vi "rsidr_core_global.vi"() -> ()   [LabVIEW 2020, in "Rohde&Schwarz RTx Oscilloscopes.lvlib"] (continued)
"Flags"=0, "Help"="Contains attributes for Spectrum Waveform settings."}, {"Level"=3, "Class Only"=FALSE, "Identifier"="RSRTX_ATTR_SPECTRUM_WAVEFORM_ENABLE", "Descriptive Name"="Spectrum Waveform Enable", "Data Type"=3, "Command"="SPEC:WAV:SPEC", "Access"=2, "Range Table"="", "Read Callback"="", "Write Callback"="", "Supported Models"="", "Instrument Options"="", "Flags"=0, "Help"="Enables or diables the indicated waveform.\n\nAvailable Repeated Capabilities:\nNone\n\nRemote-control command(s):\nSPECtrum:WAVeform:SPECtrum[:ENABle]"}, {"Level"=3, "Class Only"=FALSE, "Identifier"="RSRTX_ATTR_SPECTRUM_WAVEFORM_MINIMUM_ENABLE", "Descriptive Name"="Spectrum Waveform Minimum Enable", "Data Type"=3, "Command"="SPEC:WAV:MIN", "Access"=2, "Range Table"="", "Read Callback"="", "Write Callback"="", "Supported Models"="", "Instrument Options"="", "Flags"=0, "Help"="Enables or diables the indicated waveform.\n\nAvailable Repeated Capabilities:\nNone\n\nRemote-control command(s):\nSPECtrum:WAVeform:MINimum[:ENABle]"}, {"Level"=3, "Class Only"=FALSE, "Identifier"="RSRTX_ATTR_SPECTRUM_WAVEFORM_MAXIMUM_ENABLE", "Descriptive Name"="Spectrum Waveform Maximum Enable", "Data Type"=3, "Command"="SPEC:WAV:MAX", "Access"=2, "Range Table"="", "Read Callback"="", "Write Callback"="", "Supported Models"="", "Instrument Options"="", "Flags"=0, "Help"="Enables or diables the indicated waveform.\n\nAvailable Repeated Capabilities:\nNone\n\nRemote-control command(s):\nSPECtrum:WAVeform:MAXimum[:ENABle]"}, {"Level"=3, "Class Only"=FALSE, "Identifier"="RSRTX_ATTR_SPECTRUM_WAVEFORM_AVERAGE_ENABLE", "Descriptive Name"="Spectrum Waveform Average Enable", "Data Type"=3, "Command"="SPEC:WAV:AVER", "Access"=2, "Range Table"="", "Read Callback"="", "Write Callback"="", "Supported Models"="", "Instrument Options"="", "Flags"=0, "Help"="Enables or diables the indicated waveform.\n\nAvailable Repeated Capabilities:\nNone\n\nRemote-control command(s):\nSPECtrum:WAVeform:AVERage[:ENABle]"}, {"Level"=2, "Class Only"=TRUE, "Identifier"="", "Descriptive Name"="Time Domain", "Data Type"=0, "Command"="", "Access"=0, "Range Table"="", "Read Callback"="", "Write Callback"="", "Supported Models"="", "Instrument Options"="", "Flags"=0, "Help"="Contains attributes for Spectrum Time Domain settings."}, {"Level"=3, "Class Only"=FALSE, "Identifier"="RSRTX_ATTR_SPECTRUM_TIME_DOMAIN_POSITION", "Descriptive Name"="Spectrum Time Domain Position", "Data Type"=1, "Command"="SPEC:TIME:POS", "Access"=2, "Range Table"="", "Read Callback"="", "Write Callback"="", "Supported Models"="", "Instrument Options"="", "Flags"=0, "Help"="Sets the time position of the analyzed time range.\n\nAvailable Repeated Capabilities:\nNone\n\nRemote-control command(s):\nSPECtrum:TIME:POSition"}, {"Level"=3, "Class Only"=FALSE, "Identifier"="RSRTX_ATTR_SPECTRUM_TIME_DOMAIN_RANGE", "Descriptive Name"="Spectrum Time Domain Range", "Data Type"=1, "Command"="SPEC:TIME:RANG", "Access"=2, "Range Table"="", "Read Callback"="", "Write Callback"="", "Supported Models"="", "Instrument Options"="", "Flags"=0, "Help"="Sets the time range for the time domain diagram.\n\nAvailable Repeated Capabilities:\nNone\n\nRemote-control command(s):\nSPECtrum:TIME:RANGe"}, {"Level"=1, "Class Only"=TRUE, "Identifier"="", "Descriptive Name"="Digital Voltmeter and Counter", "Data Type"=0, "Command"="", "Access"=0, "Range Table"="", "Read Callback"="", "Write Callback"="", "Supported Models"="", "Instrument Options"="", "Flags"=0, "Help"="Contains attributes for DVM and Counter settings."}, {"Level"=2, "Class Only"=FALSE, "Identifier"="RSRTX_ATTR_DVM_ENABLE", "Descriptive Name"="DVM Enable", "Data Type"=3, "Command"="DVM{DigitalVoltmeter}:ENAB", "Access"=2, "Range Table"="", "Read Callback"="", "Write Callback"="", "Supported Models"="", "Instrument Options"="", "Flags"=0, "Help"="Enables and disables all configured voltmeter measurements.\n\nAvailable Repeated Capabilities:\nDigitalVoltmeter: DVM1, DVM2, DVM3, DVM4\r\n\nRemote-control command(s):\nDVM<m>:ENABle"}, {"Level"=2, "Class Only"=FALSE, "Identifier"="RSRTX_ATTR_DVM_SOURCE", "Descriptive Name"="DVM Source", "Data Type"=0, "Command"="DVM{DigitalVoltmeter}:SOUR", "Access"=2, "Range Table"="rsrtx_rngSource", "Read Callback"="", "Write Callback"="", "Supported Models"="", "Instrument Options"="", "Flags"=0, "Help"="Sets the measurement source for the indicated DVM measurement.\n\nAvailable Repeated Capabilities:\nDigitalVoltmeter: DVM1, DVM2, DVM3, DVM4\r\n\nRemote-control command(s):\nDVM<m>:SOURce"}, {"Level"=2, "Class Only"=FALSE, "Identifier"="RSRTX_ATTR_DVM_TYPE", "Descriptive Name"="DVM Type", "Data Type"=0, "Command"="DVM{DigitalVoltmeter}:TYPE", "Access"=2, "Range Table"="RsRtx_rngDVMType", "Read Callback"="", "Write Callback"="", "Supported Models"="", "Instrument Options"="", "Flags"=0, "Help"="Sets the measurement type for the indicated DVM measurement.\nSet OFF to disable the measurement.\n\nAvailable Repeated Capabilities:\nDigitalVoltmeter: DVM1, DVM2, DVM3, DVM4\r\n\nRemote-control command(s):\nDVM<m>:TYPE"}, {"Level"=2, "Class Only"=FALSE, "Identifier"="RSRTX_ATTR_DVM_POSITION", "Descriptive Name"="DVM Position", "Data Type"=0, "Command"="DVM{DigitalVoltmeter}:POS", "Access"=2, "Range Table"="RsRtx_rngDVMPosition", "Read Callback"="", "Write Callback"="", "Supported Models"="", "Instrument Options"="", "Flags"=0, "Help"="Sets the corner of the screen in which the measurement results are displayed.\n\nAvailable Repeated Capabilities:\nDigitalVoltmeter: DVM1, DVM2, DVM3, DVM4\r\n\nRemote-control command(s):\nDVM<m>:POSition"}, {"Level"=2, "Class Only"=FALSE, "Identifier"="RSRTX_ATTR_DVM_RESULT", "Descriptive Name"="DVM Result", "Data Type"=1, "Command"="DVM{DigitalVoltmeter}:RES?", "Access"=0, "Range Table"="", "Read Callback"="", "Write Callback"="", "Supported Models"="", "Instrument Options"="", "Flags"=0, "Help"="Returns the current value of the indicated measurement.\n\nAvailable Repeated Capabilities:\nDigitalVoltmeter: DVM1, DVM2, DVM3, DVM4\r\n\nRemote-control command(s):\nDVM<m>:RESult[:ACTual]?"}, {"Level"=2, "Class Only"=FALSE, "Identifier"="RSRTX_ATTR_DVM_RESULT_STATUS", "Descriptive Name"="DVM Result Status", "Data Type"=2, "Command"="DVM{DigitalVoltmeter}:RES:STAT?", "Access"=0, "Range Table"="", "Read Callback"="", "Write Callback"="", "Supported Models"="", "Instrument Options"="", "Flags"=0, "Help"="Returns the result value and the status of the result.\nThe status is the decimal representation of a 4-bit register value:\nBit 0 = 1: result is valid\nBit 1 = 1: no result available\nBit 2 = 1: clipping occurs\nBit 3 = 1: no period found\n\nAvailable Repeated Capabilities:\nDigitalVoltmeter: DVM1, DVM2, DVM3, DVM4\r\n\nRemote-control command(s):\nDVM<m>:RESult[:ACTual]:STATus?"}, {"Level"=2, "Class Only"=TRUE, "Identifier"="", "Descriptive Name"="Counter", "Data Type"=0, "Command"="", "Access"=0, "Range Table"="", "Read Callback"="", "Write Callback"="", "Supported Models"="", "Instrument Options"="", "Flags"=0, "Help"="Contains attributes for Counter Settings and Results."}, {"Level"=3, "Class Only"=FALSE, "Identifier"="RSRTX_ATTR_COUNTER_ENABLE", "Descriptive Name"="Counter Enable", "Data Type"=3, "Command"="TCO:ENAB", "Access"=2, "Range Table"="", "Read Callback"="", "Write Callback"="", "Supported Models"="", "Instrument Options"="", "Flags"=0, "Help"="Enables or disables the trigger counter measurements.\n\nAvailable Repeated Capabilities:\nNone\n\nRemote-control command(s):\nTCOunter:ENABle"}, {"Level"=3, "Class Only"=FALSE, "Identifier"="RSRTX_ATTR_COUNTER_FREQUENCY", "Descriptive Name"="Counter Frequency", "Data Type"=1, "Command"="TCO:RES:FREQ?", "Access"=0, "Range Table"="", "Read Callback"="", "Write Callback"="", "Supported Models"="", "Instrument Options"="", "Flags"=0, "Help"="Returns the frequency of the trigger source.\n\nAvailable Repeated Capabilities:\nNone\n\nRemote-control command(s):\nTCOunter:RESult[:ACTual]:FREQuency?"}, {"Level"=3, "Class Only"=FALSE, "Identifier"="RSRTX_ATTR_COUNTER_PERIOD", "Descriptive Name"="Counter Period", "Data Type"=1, "Command"="TCO:RES:PER?", "Access"=0, "Range Table"="", "Read Callback"="", "Write Callback"="", "Supported Models"="", "Instrument Options"="", "Flags"=0, "Help"="Returns the period of the trigger source.\n\nAvailable Repeated Capabilities:\nNone\n\nRemote-control command(s):\nTCOunter:RESult[:ACTual]:PERiod?"}, {"Level"=3, "Class Only"=FALSE, "Identifier"="RSRTX_ATTR_COUNTER_SOURCE", "Descriptive Name"="Counter Source", "Data Type"=0, "Command"="TCO:SOUR", "Access"=2, "Range Table"="RsRtx_rngCounterSource", "Read Callback"="", "Write Callback"="", "Supported Models"="", "Instrument Options"="", "Flags"=0, "Help"="Sets the measurement source for the counter.\n\nAvailable Repeated Capabilities:\nNone\n\nRemote-control command(s):\nTCOunter:SOURce"}, {"Level"=1, "Class Only"=TRUE, "Identifier"="", "Descriptive Name"="Bode Plot", "Data Type"=0, "Command"="", "Access"=0, "Range Table"="", "Read Callback"="", "Write Callback"="", "Supported Models"="", "Instrument Options"="", "Flags"=0, "Help"="This class contains methods for the Bode Plot application (option R&S RTM-K36)."}, {"Level"=2, "Class Only"=FALSE, "Identifier"="RSRTX_ATTR_BODE_PLOT_ENABLE", "Descriptive Name"="Bode Plot Enable", "Data Type"=3, "Command"="BPL:ENAB", "Access"=2, "Range Table"="", "Read Callback"="", "Write Callback"="", "Supported Models"="", "Instrument Options"="K36", "Flags"=0, "Help"="Enables the Bode plot diagram.\n\nAvailable Repeated Capabilities:\nNone\n\nRemote-control command(s):\nBPLot:ENABle"}, {"Level"=2, "Class Only"=FALSE, "Identifier"="RSRTX_ATTR_BODE_PLOT_START_FREQUENCY", "Descriptive Name"="Bode Plot Start Frequency", "Data Type"=1, "Command"="BPL:FREQ:STAR", "Access"=2, "Range Table"="RsRtx_rngBodePlotStartFrequency", "Read Callback"="", "Write Callback"="", "Supported Models"="", "Instrument Options"="K36", "Flags"=0, "Help"="Sets the start frequency of the sweep for the Bode plot.\n\nAvailable Repeated Capabilities:\nNone\n\nRemote-control command(s):\nBPLot:FREQuency:STARt"}, {"Level"=2, "Class Only"=FALSE, "Identifier"="RSRTX_ATTR_BODE_PLOT_STOP_FREQUENCY", "Descriptive Name"="Bode Plot Stop Frequency", "Data Type"=1, "Command"="BPL:FREQ:STOP", "Access"=2, "Range Table"="RsRtx_rngBodePlotStopFrequency", "Read Callback"="", "Write Callback"="", "Supported Models"="", "Instrument Options"="K36", "Flags"=0, "Help"="Sets the stop frequency of the sweep for the Bode plot.\n\nAvailable Repeated Capabilities:\nNone\n\nRemote-control command(s):\nBPLot:FREQuency:STOP"}, {"Level"=2, "Class Only"=FALSE, "Identifier"="RSRTX_ATTR_BODE_PLOT_AUTOSCALE", "Descriptive Name"="Bode Plot Autoscale", "Data Type"=4, "Command"="BPL:AUT", "Access"=1, "Range Table"="", "Read Callback"="", "Write Callback"="", "Supported Models"="", "Instrument Options"="", "Flags"=0, "Help"="Sets the start and stop frequencies for the Bode plot automatically.\n\nAvailable Repeated Capabilities:\nNone\n\nRemote-control command(s):\nBPLot:AUToscale"}, {"Level"=2, "Class Only"=FALSE, "Identifier"="RSRTX_ATTR_BODE_PLOT_INPUT_CHANNEL", "Descriptive Name"="Bode Plot Input Channel", "Data Type"=0, "Command"="BPL:INP", "Access"=2, "Range Table"="RsRtx_rngBodeSourceChannel", "Read Callback"="", "Write Callback"="", "Supported Models"="", "Instrument Options"="", "Flags"=0, "Help"="Selects the channel for the input signal of the DUT.\n\nAvailable Repeated Capabilities:\nNone\n\nRemote-control command(s):\nBPLot:INPut[:SOURce]"}, {"Level"=2, "Class Only"=FALSE, "Identifier"="RSRTX_ATTR_BODE_PLOT_OUTPUT_CHANNEL", "Descriptive Name"="Bode Plot Output Channel", "Data Type"=0, "Command"="BPL:OUTP", "Access"=2, "Range Table"="RsRtx_rngBodeSourceChannel", "Read Callback"="", "Write Callback"="", "Supported Models"="", "Instrument Options"="", "Flags"=0, "Help"="Selects the channel for the output signal of the DUT.\n\nAvailable Repeated Capabilities:\nNone\n\nRemote-control command(s):\nBPLot:OUTPut[:SOURce]"}, {"Level"=2, "Class Only"=FALSE, "Identifier"="RSRTX_ATTR_BODE_PLOT_GAIN_ENABLE", "Descriptive Name"="Bode Plot Gain Enable", "Data Type"=3, "Command"="BPL:GAIN:ENAB", "Access"=2, "Range Table"="", "Read Callback"="", "Write Callback"="", "Supported Models"="", "Instrument Options"="", "Flags"=0, "Help"="Enables the gain waveform for the Bode plot.\n\nAvailable Repeated Capabilities:\nNone\n\nRemote-control command(s):\nBPLot:GAIN:ENABle"}, {"Level"=2, "Class Only"=FALSE, "Identifier"="RSRTX_ATTR_BODE_PLOT_GAIN_POSITION", "Descriptive Name"="Bode Plot Gain Position", "Data Type"=1, "Command"="BPL:GAIN:POS", "Access"=2, "Range Table"="RsRtx_rngBodeGainPosition", "Read Callback"="", "Write Callback"="", "Supported Models"="", "Instrument Options"="", "Flags"=0, "Help"="Sets the vertical position of the gain waveform in divisions.\n\nAvailable Repeated Capabilities:\nNone\n\nRemote-control command(s):\nBPLot:GAIN:POSition"}, {"Level"=2, "Class Only"=FALSE, "Identifier"="RSRTX_ATTR_BODE_PLOT_GAIN_SCALE", "Descriptive Name"="Bode Plot Gain Scale", "Data Type"=1, "Command"="BPL:GAIN:SCAL", "Access"=2, "Range Table"="RsRtx_rngBodeGainScale", "Read Callback"="", "Write Callback"="", "Supported Models"="", "Instrument Options"="K36", "Flags"=0, "Help"="Sets the vertical scale for the gain waveform.\n\nAvailable Repeated Capabilities:\nNone\n\nRemote-control command(s):\nBPLot:GAIN:SCALe"}, {"Level"=2, "Class Only"=FALSE, "Identifier"="RSRTX_ATTR_BODE_PLOT_PHASE_ENABLE", "Descriptive Name"="Bode Plot Phase Enable", "Data Type"=3, "Command"="BPL:PHAS:ENAB?", "Access"=0, "Range Table"="", "Read Callback"="", "Write Callback"="", "Supported Models"="", "Instrument Options"="", "Flags"=0, "Help"="Enables the phase waveform for the Bode plot.\n\nAvailable Repeated Capabilities:\nNone\n\nRemote-control command(s):\nBPLot:PHASe:ENABle?"}, {"Level"=2, "Class Only"=FALSE, "Identifier"="RSRTX_ATTR_BODE_PLOT_PHASE_POSITION", "Descriptive Name"="Bode Plot Phase Position", "Data Type"=1, "Command"="BPL:PHAS:POS?", "Access"=0, "Range Table"="RsRtx_rngBodePhasePosition", "Read Callback"="", "Write Callback"="", "Supported Models"="", "Instrument Options"="", "Flags"=0, "Help"="Sets the vertical position of the phase waveform in divisions.\n\nAvailable Repeated Capabilities:\nNone\n\nRemote-control command(s):\nBPLot:PHASe:POSition?"}, {"Level"=2, "Class Only"=FALSE, "Identifier"="RSRTX_ATTR_BODE_PLOT_PHASE_SCALE", "Descriptive Name"="Bode Plot Phase Scale", "Data Type"=1, "Command"="BPL:PHAS:SCAL?", "Access"=0, "Range Table"="RsRtx_rngBodePhaseScale", "Read Callback"="", "Write Callback"="", "Supported Models"="", "Instrument Options"="K36", "Flags"=0, "Help"="Sets the vertical scale for the phase waveform.\n\nAvailable Repeated Capabilities:\nNone\n\nRemote-control command(s):\nBPLot:PHASe:SCALe?"}, {"Level"=2, "Class Only"=FALSE, "Identifier"="RSRTX_ATTR_BODE_PLOT_AMPLITUDE_ENABLE", "Descriptive Name"="Bode Plot Amplitude Enable", "Data Type"=3, "Command"="BPL:AMPL:ENAB", "Access"=2, "Range Table"="", "Read Callback"="", "Write Callback"="", "Supported Models"="", "Instrument Options"="K36", "Flags"=0, "Help"="Enables the amplitude waveform for the Bode plot.\n\nAvailable Repeated Capabilities:\nNone\n\nRemote-control command(s):\nBPLot:AMPLitude:ENABle"}, {"Level"=2, "Class Only"=FALSE, "Identifier"="RSRTX_ATTR_BODE_PLOT_AMPLITUDE_POSITION", "Descriptive Name"="Bode Plot Amplitude Position", "Data Type"=1, "Command"="BPL:AMPL:POS", "Access"=2, "Range Table"="RsRtx_rngBodeAmplitudePosition", "Read Callback"="", "Write Callback"="", "Supported Models"="", "Instrument Options"="K36", "Flags"=0, "Help"="Sets the vertical position of the amplitude waveform in divisions.\n\nAvailable Repeated Capabilities:\nNone\n\nRemote-control command(s):\nBPLot:AMPLitude:POSition"}, {"Level"=2, "Class Only"=FALSE, "Identifier"="RSRTX_ATTR_BODE_PLOT_AMPLITUDE_SCALE", "Descriptive Name"="Bode Plot Amplitude Scale", "Data Type"=1, "Command"="BPL:AMPL:SCAL", "Access"=2, "Range Table"="RsRtx_rngBodeAmplitudeScale", "Read Callback"="", "Write Callback"="", "Supported Models"="", "Instrument Options"="K36", "Flags"=0, "Help"="Sets the vertical scale for the amplitude waveform.\n\nAvailable Repeated Capabilities:\nNone\n\nRemote-control command(s):\nBPLot:AMPLitude:SCALe"}, {"Level"=2, "Class Only"=FALSE, "Identifier"="RSRTX_ATTR_START_BODE_PLOT_MEASUREMENT", "Descriptive Name"="Start Bode Plot Measurement", "Data Type"=4, "Command"="BPL:STAT RUN", "Access"=1, "Range Table"="", "Read Callback"="", "Write Callback"="", "Supported Models"="", "Instrument Options"="K36", "Flags"=0, "Help"="Starts the Bode plot measurement.\n\nAvailable Repeated Capabilities:\nNone\n\nRemote-control command(s):\nBPLot:STATe RUN"}, {"Level"=2, "Class Only"=FALSE, "Identifier"="RSRTX_ATTR_STOP_BODE_PLOT_MEASUREMENT", "Descriptive Name"="Stop Bode Plot Measurement", "Data Type"=4, "Command"="BPL:STAT STOP", "Access"=1, "Range Table"="", "Read Callback"="", "Write Callback"="", "Supported Models"="", "Instrument Options"="K36", "Flags"=0, "Help"="Stops the Bode plot measurement.\n\nAvailable Repeated Capabilities:\nNone\n\nRemote-control command(s):\nBPLot:STATe STOP"}, {"Level"=2, "Class Only"=FALSE, "Identifier"="RSRTX_ATTR_BODE_PLOT_MEASUREMENT_STATE", "Descriptive Name"="Bode Plot Measurement State", "Data Type"=0, "Command"="BPL:STAT", "Access"=2, "Range Table"="RsRtx_rngBodePlotMeasurementState", "Read Callback"="", "Write Callback"="", "Supported Models"="", "Instrument Options"="K36", "Flags"=0, "Help"="Starts or stops the Bode plot measurement.\n\nAvailable Repeated Capabilities:\nNone\n\nRemote-control command(s):\nBPLot:STATe"}, {"Level"=2, "Class Only"=FALSE, "Identifier"="RSRTX_ATTR_BODE_PLOT_REPEATED_MEASUREMENT_ENABLE", "Descriptive Name"="Bode Plot Repeated Measurement Enable", "Data Type"=3, "Command"="BPL:REP", "Access"=2, "Range Table"="", "Read Callback"="", "Write Callback"="", "Supported Models"="", "Instrument Options"="K36", "Flags"=0, "Help"="Repeats the measurement, using the same parameters.\n\nAvailable Repeated Capabilities:\nNone\n\nRemote-control command(s):\nBPLot:REPeat"}, {"Level"=2, "Class Only"=FALSE, "Identifier"="RSRTX_ATTR_BODE_PLOT_RESET", "Descriptive Name"="Bode Plot Reset", "Data Type"=4, "Command"="BPL:RES", "Access"=1, "Range Table"="", "Read Callback"="", "Write Callback"="", "Supported Models"="", "Instrument Options"="", "Flags"=0, "Help"="Deletes all test results.\n\nAvailable Repeated Capabilities:\nNone\n\nRemote-control command(s):\nBPLot:RESet"}, {"Level"=2, "Class Only"=FALSE, "Identifier"="RSRTX_ATTR_BODE_PLOT_AMPLITUDE_MODE", "Descriptive Name"="Bode Plot Amplitude Mode", "Data Type"=0, "Command"="BPL:AMPL:MODE", "Access"=2, "Range Table"="RsRtx_rngBodeAmplitudeMode", "Read Callback"="", "Write Callback"="", "Supported Models"="", "Instrument Options"="K36", "Flags"=0, "Help"="Sets the amplitude mode.\n\nAvailable Repeated Capabilities:\nNone\n\nRemote-control command(s):\nBPLot:AMPLitude:MODE"}, {"Level"=2, "Class Only"=FALSE, "Identifier"="RSRTX_ATTR_BODE_PLOT_POINTS_PER_DECADE", "Descriptive Name"="Bode Plot Points Per Decade", "Data Type"=0, "Command"="BPL:POIN:LOG", "Access"=2, "Range Table"="RsRtx_rngBodePointsPerDecade", "Read Callback"="", "Write Callback"="", "Supported Models"="", "Instrument Options"="K36", "Flags"=0, "Help"="Sets the number of points per decade that are measured.\n\nAvailable Repeated Capabilities:\nNone\n\nRemote-control command(s):\nBPLot:POINts:LOGarithmic"}, {"Level"=2, "Class Only"=FALSE, "Identifier"="RSRTX_ATTR_BODE_PLOT_MEASUREMENT_POINTS_DISPLAY_ENABLE", "Descriptive Name"="Bode Plot Measurement Points Display Enable", "Data Type"=3, "Command"="BPL:MEAS:POIN", "Access"=2, "Range Table"="", "Read Callback"="", "Write Callback"="", "Supported Models"="", "Instrument Options"="K36", "Flags"=0, "Help"="Enables the display of the measurement points in the bode plot.\n\nAvailable Repeated Capabilities:\nNone\n\nRemote-control command(s):\nBPLot:MEASurement:POINt[:DISPLAY]"}, {"Level"=2, "Class Only"=FALSE, "Identifier"="RSRTX_ATTR_BODE_PLOT_MEASUREMENT_DELAY", "Descriptive Name"="Bode Plot Measurement Delay", "Data Type"=1, "Command"="BPL:MEAS:DEL", "Access"=2, "Range Table"="RsRtx_rngBodeMeasurementDelay", "Read Callback"="", "Write Callback"="", "Supported Models"="", "Instrument Options"="", "Flags"=0, "Help"="Sets a time delay, that the system waits before measuring the next point of the bode plot.\n\nAvailable Repeated Capabilities:\nNone\n\nRemote-control command(s):\nBPLot:MEASurement:DELay"}, {"Level"=2, "Class Only"=FALSE, "Identifier"="RSRTX_ATTR_BODE_PLOT_EXPORT_NAME", "Descriptive Name"="Bode Plot Export Name", "Data Type"=2, "Command"="BPL:EXP:NAME", "Access"=2, "Range Table"="", "Read Callback"="", "Write Callback"="", "Supported Models"="", "Instrument Options"="K36", "Flags"=0, "Help"="Path and file name to save Bode plot export data. File format is CSV\n\nAvailable Repeated Capabilities:\nNone\n\nRemote-control command(s):\nBPLot:EXPort:NAME"}, {"Level"=2, "Class Only"=FALSE, "Identifier"="RSRTX_ATTR_BODE_PLOT_EXPORT_SAVE", "Descriptive Name"="Bode Plot Export Save", "Data Type"=4, "Command"="BPL:EXP:SAVE", "Access"=1, "Range Table"="", "Read Callback"="", "Write Callback"="", "Supported Models"="", "Instrument Options"="K36", "Flags"=0, "Help"="Saves the acquisition timestamps table to the file that is defined by RSRTX_ATTR_BODE_PLOT_EXPORT_NAME.\n\nAvailable Repeated Capabilities:\nNone\n\nRemote-control command(s):\nBPLot:EXPort:SAVE"}, {"Level"=2, "Class Only"=TRUE, "Identifier"="", "Descriptive Name"="Amplitude Profile", "Data Type"=0, "Command"="", "Access"=0, "Range Table"="", "Read Callback"="", "Write Callback"="", "Supported Models"="", "Instrument Options"="", "Flags"=0, "Help"="This class contains methods for configuring the points in the Bode plot amplitude profile."}, {"Level"=3, "Class Only"=FALSE, "Identifier"="RSRTX_ATTR_BODE_PLOT_AMPLITUDE_PROFILE_POINTS", "Descriptive Name"="Bode Plot Amplitude Profile Points", "Data Type"=1, "Command"="BPL:AMPL:PROF:COUN", "Access"=2, "Range Table"="RsRtx_rngBodeAmplitudeProfilePoints", "Read Callback"="", "Write Callback"="", "Supported Models"="", "Instrument Options"="K36", "Flags"=0, "Help"="Sets the number of different points that you can define for the amplitude profile.\n\nAvailable Repeated Capabilities:\nNone\n\nRemote-control command(s):\nBPLot:AMPLitude:PROFile:COUNt"}, {"Level"=3, "Class Only"=FALSE, "Identifier"="RSRTX_ATTR_BODE_PLOT_AMPLITUDE_PROFILE_POINT_AMPLITUDE", "Descriptive Name"="Bode Plot Amplitude Profile Point Amplitude", "Data Type"=1, "Command"="BPL:AMPL:PROF:POIN{ProfilePoint}:AMPL", "Access"=2, "Range Table"="", "Read Callback"="", "Write Callback"="", "Supported Models"="", "Instrument Options"="K36", "Flags"=0, "Help"="Sets the amplitude of the specified point of the amplitude profile.\n\nAvailable Repeated Capabilities:\nProfilePoint: Point1, Point2, Point3, Point4, Point5, Point6, Point7, Point8, Point9, Point10, Point11, Point12, Point13, Point14, Point15, Point16\r\n\nRemote-control command(s):\nBPLot:AMPLitude:PROFile:POINt<n>:AMPLitude"}, {"Level"=3, "Class Only"=FALSE, "Identifier"="RSRTX_ATTR_BODE_PLOT_AMPLITUDE_PROFILE_POINT_FREQUENCY", "Descriptive Name"="Bode Plot Amplitude Profile Point Frequency", "Data Type"=1, "Command"="BPL:AMPL:PROF:POIN{ProfilePoint}:FREQ", "Access"=2, "Range Table"="", "Read Callback"="", "Write Callback"="", "Supported Models"="", "Instrument Options"="K36", "Flags"=0, "Help"="Sets the frequency of the specified point of the amplitude profile.\n\nAvailable Repeated Capabilities:\nProfilePoint: Point1, Point2, Point3, Point4, Point5, Point6, Point7, Point8, Point9, Point10, Point11, Point12, Point13, Point14, Point15, Point16\r\n\nRemote-control command(s):\nBPLot:AMPLitude:PROFile:POINt<n>:FREQuency"}, {"Level"=2, "Class Only"=TRUE, "Identifier"="", "Descriptive Name"="Marker", "Data Type"=0, "Command"="", "Access"=0, "Range Table"="", "Read Callback"="", "Write Callback"="", "Supported Models"="", "Instrument Options"="", "Flags"=0, "Help"="This class contains methods for the Bode plot marker table."}, {"Level"=3, "Class Only"=FALSE, "Identifier"="RSRTX_ATTR_BODE_PLOT_MARKER_FREQUENCY", "Descriptive Name"="Bode Plot Marker Frequency", "Data Type"=1, "Command"="BPL:MARK{BodeMarker}:FREQ", "Access"=2, "Range Table"="", "Read Callback"="", "Write Callback"="", "Supported Models"="", "Instrument Options"="K36", "Flags"=0, "Help"="Returns the frequency for the specified marker.\n\nAvailable Repeated Capabilities:\nBodeMarker: BodeMark1, BodeMark2\r\n\nRemote-control command(s):\nBPLot:MARKer<m>:FREQuency"}, {"Level"=3, "Class Only"=FALSE, "Identifier"="RSRTX_ATTR_BODE_PLOT_MARKER_GAIN", "Descriptive Name"="Bode Plot Marker Gain", "Data Type"=1, "Command"="BPL:MARK{BodeMarker}:GAIN?", "Access"=0, "Range Table"="", "Read Callback"="", "Write Callback"="", "Supported Models"="", "Instrument Options"="K36", "Flags"=0, "Help"="Returns the gain for the specified marker.\n\nAvailable Repeated Capabilities:\nBodeMarker: BodeMark1, BodeMark2\r\n\nRemote-control command(s):\nBPLot:MARKer<m>:GAIN?"}, {"Level"=3, "Class Only"=FALSE, "Identifier"="RSRTX_ATTR_BODE_PLOT_MARKER_PHASE", "Descriptive Name"="Bode Plot Marker Phase", "Data Type"=1, "Command"="BPL:MARK{BodeMarker}:PHAS?", "Access"=0, "Range Table"="", "Read Callback"="", "Write Callback"="", "Supported Models"="", "Instrument Options"="K36", "Flags"=0, "Help"="Returns the phase value for the specified marker.\n\nAvailable Repeated Capabilities:\nBodeMarker: BodeMark1, BodeMark2\r\n\nRemote-control command(s):\nBPLot:MARKer<m>:PHASe?"}, {"Level"=3, "Class Only"=FALSE, "Identifier"="RSRTX_ATTR_BODE_PLOT_MARKER_INDEX", "Descriptive Name"="Bode Plot Marker Index", "Data Type"=1, "Command"="BPL:MARK{BodeMarker}:IND", "Access"=2, "Range Table"="", "Read Callback"="", "Write Callback"="", "Supported Models"="", "Instrument Options"="K36", "Flags"=0, "Help"="Returns the index for the specified marker.\n\nAvailable Repeated Capabilities:\nBodeMarker: BodeMark1, BodeMark2\r\n\nRemote-control command(s):\nBPLot:MARKer<m>:INDex"}, {"Level"=3, "Class Only"=FALSE, "Identifier"="RSRTX_ATTR_BODE_PLOT_MARKER_FREQUENCY_DIFFERENCE", "Descriptive Name"="Bode Plot Marker Frequency Difference", "Data Type"=1, "Command"="BPL:MARK:DIFF:FREQ?", "Access"=0, "Range Table"="", "Read Callback"="", "Write Callback"="", "Supported Models"="", "Instrument Options"="K36", "Flags"=0, "Help"="Returns the delta value of the frequency between the two markers.\n\nAvailable Repeated Capabilities:\nNone\n\nRemote-control command(s):\nBPLot:MARKer<m>:DIFFerence:FREQ?"}, {"Level"=3, "Class Only"=FALSE, "Identifier"="RSRTX_ATTR_BODE_PLOT_MARKER_GAIN_DIFFERENCE", "Descriptive Name"="Bode Plot Marker Gain Difference", "Data Type"=1, "Command"="BPL:MARK:DIFF:GAIN?", "Access"=0, "Range Table"="", "Read Callback"="", "Write Callback"="", "Supported Models"="", "Instrument Options"="K36", "Flags"=0, "Help"="Returns the delta value of the gain between the two markers.\n\nAvailable Repeated Capabilities:\nNone\n\nRemote-control command(s):\nBPLot:MARKer<m>:DIFFerence:GAIN?"}, {"Level"=3, "Class Only"=FALSE, "Identifier"="RSRTX_ATTR_BODE_PLOT_MARKER_PHASE_DIFFERENCE", "Descriptive Name"="Bode Plot Marker Phase Difference", "Data Type"=1, "Command"="BPL:MARK:DIFF:PHAS?", "Access"=0, "Range Table"="", "Read Callback"="", "Write Callback"="", "Supported Models"="", "Instrument Options"="K36", "Flags"=0, "Help"="Returns the delta value of the phase between the two markers.\n\nAvailable Repeated Capabilities:\nNone\n\nRemote-control command(s):\nBPLot:MARKer<m>:DIFFerence:PHASe?"}, {"Level"=3, "Class Only"=FALSE, "Identifier"="RSRTX_ATTR_RESET_BODE_PLOT_MARKERS", "Descriptive Name"="Reset Bode Plot Markers", "Data Type"=4, "Command"="BPL:MARK:SSCR", "Access"=1, "Range Table"="", "Read Callback"="", "Write Callback"="", "Supported Models"="", "Instrument Options"="K36", "Flags"=0, "Help"="Resets the markers to their initial positions. This is helpful if the markers have disappeared from the display or need to be moved for a larger distance.\n\nAvailable Repeated Capabilities:\nNone\n\nRemote-control command(s):\nBPLot:MARKer<m>:SSCReen"}, {"Level"=2, "Class Only"=TRUE, "Identifier"="", "Descriptive Name"="Results", "Data Type"=0, "Command"="", "Access"=0, "Range Table"="", "Read Callback"="", "Write Callback"="", "Supported Models"="", "Instrument Options"="", "Flags"=0, "Help"="This class contains methods for accessing the results of Bode plot measurements."}, {"Level"=1, "Class Only"=TRUE, "Identifier"="", "Descriptive Name"="Generator", "Data Type"=0, "Command"="", "Access"=0, "Range Table"="", "Read Callback"="", "Write Callback"="", "Supported Models"="", "Instrument Options"="", "Flags"=0, "Help"="The R&S RTO includes an integrated waveform generator which can generate input signals and patterns during testing.\nYou can setup and output two waveform generators and a pattern generator. It is possible to couple and synchronize the settings of the different generators and enable them on a trigger signal. With each of the waveform generators, one can output simple functions, modulated sine waveform, arbitrary waveforms and sweep waveforms."}, {"Level"=2, "Class Only"=TRUE, "Identifier"="", "Descriptive Name"="Waveform Generator", "Data Type"=0, "Command"="", "Access"=0, "Range Table"="", "Read Callback"="", "Write Callback"="", "Supported Models"="", "Instrument Options"="", "Flags"=0, "Help"="Integrated waveform generator which can generate input signals."}, {"Level"=3, "Class Only"=TRUE, "Identifier"="", "Descriptive Name"="Function Generator", "Data Type"=0, "Command"="", "Access"=0, "Range Table"="", "Read Callback"="", "Write Callback"="", "Supported Models"="", "Instrument Options"="", "Flags"=0, "Help"="The R&S RTO function generator can generate input signals during testing. These signals can be used for example, when testing circuits."}, {"Level"=4, "Class Only"=FALSE, "Identifier"="RSRTX_ATTR_WAVEFORM_GENERATOR_FUNCTION_TYPE", "Descriptive Name"="Waveform Generator Function Type", "Data Type"=0, "Command"="WGEN:FUNC", "Access"=2, "Range Table"="RsRtx_rngWaveformGeneratorFunctionType", "Read Callback"="", "Write Callback"="", "Supported Models"="", "Instrument Options"="", "Flags"=0, "Help"="Sets the type of waveform to be generated for the function generator.\n\nAvailable Repeated Capabilities:\nNone\n\nRemote-control command(s):\nWGENerator:FUNCtion"}, {"Level"=4, "Class Only"=FALSE, "Identifier"="RSRTX_ATTR_WAVEFORM_GENERATOR_FREQUENCY", "Descriptive Name"="Waveform Generator Frequency", "Data Type"=1, "Command"="WGEN:FREQ", "Access"=2, "Range Table"="", "Read Callback"="", "Write Callback"="", "Supported Models"="", "Instrument Options"="", "Flags"=0, "Help"="Sets the frequency of the waveform. The available frequency range depends on the selected function type.\n\nAvailable Repeated Capabilities:\nNone\n\nRemote-control command(s):\nWGENerator:FREQuency"}, {"Level"=4, "Class Only"=FALSE, "Identifier"="RSRTX_ATTR_WAVEFORM_GENERATOR_PULSE_DUTY_CYCLE", "Descriptive Name"="Waveform Generator Pulse Duty Cycle", "Data Type"=1, "Command"="WGEN:FUNC:PULS:DCYC", "Access"=2, "Range Table"="RsRtx_rngWaveformGeneratorDutyCycle", "Read Callback"="", "Write Callback"="", "Supported Models"="", "Instrument Options"="", "Flags"=0, "Help"="Sets the duty cycle for a square waveform. The duty cycle expresses for what percentage of the period, the signal state is high.\n\nAvailable Repeated Capabilities:\nNone\n\nRemote-control command(s):\nWGENerator:FUNCtion:PULSe:DCYCle"}, {"Level"=4, "Class Only"=FALSE, "Identifier"="RSRTX_ATTR_WAVEFORM_GENERATOR_PULSE_EDGE_TIME", "Descriptive Name"="Waveform Generator Pulse Edge Time", "Data Type"=1, "Command"="WGEN:FUNC:PULS:ETIM", "Access"=2, "Range Table"="", "Read Callback"="", "Write Callback"="", "Supported Models"="", "Instrument Options"="", "Flags"=0, "Help"="Configures pulse edge time.\n\nAvailable Repeated Capabilities:\nNone\n\nRemote-control command(s):\nWGENerator:FUNCtion:PULSe:ETIMe"}, {"Level"=4, "Class Only"=FALSE, "Identifier"="RSRTX_ATTR_WAVEFORM_GENERATOR_RAMP_POLARITY", "Descriptive Name"="Waveform Generator Ramp Polarity", "Data Type"=0, "Command"="WGEN:FUNC:RAMP:POL", "Access"=2, "Range Table"="rsrtx_rngPolarity", "Read Callback"="", "Write Callback"="", "Supported Models"="", "Instrument Options"="", "Flags"=0, "Help"="Configures the ramp waveform polarity.\n\nAvailable Repeated Capabilities:\nNone\n\nRemote-control command(s):\nWGENerator:FUNCtion:RAMP:POLarity"}, {"Level"=4, "Class Only"=FALSE, "Identifier"="RSRTX_ATTR_WAVEFORM_GENERATOR_EXPONENTIAL_POLARITY", "Descriptive Name"="Waveform Generator Exponential Polarity", "Data Type"=0, "Command"="WGEN:FUNC:EXP:POL", "Access"=2, "Range Table"="rsrtx_rngPolarity", "Read Callback"="", "Write Callback"="", "Supported Models"="", "Instrument Options"="", "Flags"=0, "Help"="Configures the exponential waveform polarity.\n\nAvailable Repeated Capabilities:\nNone\n\nRemote-control command(s):\nWGENerator:FUNCtion:EXPonential:POLarity"}, {"Level"=4, "Class Only"=FALSE, "Identifier"="RSRTX_ATTR_WAVEFORM_GENERATOR_TRIANGLE_SYMMETRY", "Descriptive Name"="Waveform Generator Triangle Symmetry", "Data Type"=1, "Command"="WGEN:TRI:SYMM", "Access"=2, "Range Table"="RsRtx_rngTriangleSymmetry", "Read Callback"="", "Write Callback"="", "Supported Models"="", "Instrument Options"="", "Flags"=0, "Help"="Sets the symmetry for the triangle waveform. 50% defines symmetric triangles. Values <50% define triangles with steeper rising edge leaned to the left. Values >50% define triangles with steeper falling edge leaned to the right.\n\nAvailable Repeated Capabilities:\nNone\n\nRemote-control command(s):\nWGENerator:TRIangle:SYMMetry"}, {"Level"=3, "Class Only"=TRUE, "Identifier"="", "Descriptive Name"="Modulation", "Data Type"=0, "Command"="", "Access"=0, "Range Table"="", "Read Callback"="", "Write Callback"="", "Supported Models"="", "Instrument Options"="", "Flags"=0, "Help"="Modulation is when properties of an original periodic waveform, the carrier signal, are varied according to a second modulating signal. The type of modulation used determines which properties are changed."}, {"Level"=4, "Class Only"=FALSE, "Identifier"="RSRTX_ATTR_WAVEFORM_GENERATOR_MODULATION_ENABLED", "Descriptive Name"="Waveform Generator Modulation Enabled", "Data Type"=3, "Command"="WGEN:MOD", "Access"=2, "Range Table"="", "Read Callback"="", "Write Callback"="", "Supported Models"="", "Instrument Options"="", "Flags"=0, "Help"="Enables the waveform modulation.\n\nAvailable Repeated Capabilities:\nNone\n\nRemote-control command(s):\nWGENerator:MODulation[:ENABLE]"}, {"Level"=4, "Class Only"=FALSE, "Identifier"="RSRTX_ATTR_WAVEFORM_GENERATOR_MODULATION_TYPE", "Descriptive Name"="Waveform Generator Modulation Type", "Data Type"=0, "Command"="WGEN:MOD:TYPE", "Access"=2, "Range Table"="RsRtx_rngWaveformGeneratorModulationType", "Read Callback"="", "Write Callback"="", "Supported Models"="", "Instrument Options"="", "Flags"=0, "Help"="Sets the modulation type.\n\nAvailable Repeated Capabilities:\nNone\n\nRemote-control command(s):\nWGENerator:MODulation:TYPE"}, {"Level"=4, "Class Only"=FALSE, "Identifier"="RSRTX_ATTR_WAVEFORM_GENERATOR_MODULATION_FUNCTION_TYPE", "Descriptive Name"="Waveform Generator Modulation Function Type", "Data Type"=0, "Command"="WGEN:MOD:FUNC", "Access"=2, "Range Table"="RsRtx_rngWaveformGeneratorModulationFunctionType", "Read Callback"="", "Write Callback"="", "Supported Models"="", "Instrument Options"="", "Flags"=0, "Help"="Sets the function type of modulation.\n\nAvailable Repeated Capabilities:\nNone\n\nRemote-control command(s):\nWGENerator:MODulation:FUNCtion"}, {"Level"=4, "Class Only"=FALSE, "Identifier"="RSRTX_ATTR_WAVEFORM_GENERATOR_MODULATION_RAMP_POLARITY", "Descriptive Name"="Waveform Generator Modulation Ramp Polarity", "Data Type"=0, "Command"="WGEN:MOD:RAMP:POL", "Access"=2, "Range Table"="rsrtx_rngPolarity", "Read Callback"="", "Write Callback"="", "Supported Models"="", "Instrument Options"="", "Flags"=0, "Help"="Configures the ramp waveform polarity.\n\nAvailable Repeated Capabilities:\nNone\n\nRemote-control command(s):\nWGENerator:MODulation:RAMP:POLarity"}, {"Level"=4, "Class Only"=TRUE, "Identifier"="", "Descriptive Name"="AM", "Data Type"=0, "Command"="", "Access"=0, "Range Table"="", "Read Callback"="", "Write Callback"="", "Supported Models"="", "Instrument Options"="", "Flags"=0, "Help"="For amplitude modulation (AM), the amplitude of the carrier signal is varied according to the modulation signal."}, {"Level"=5, "Class Only"=FALSE, "Identifier"="RSRTX_ATTR_WAVEFORM_GENERATOR_AM_MODULATION_FREQUENCY", "Descriptive Name"="Waveform Generator AM Modulation Frequency", "Data Type"=1, "Command"="WGEN:MOD:AM:FREQ", "Access"=2, "Range Table"="", "Read Callback"="", "Write Callback"="", "Supported Models"="", "Instrument Options"="", "Flags"=0, "Help"="Sets the frequency of the modulation waveform for amplitude modulation.\n\nAvailable Repeated Capabilities:\nNone\n\nRemote-control command(s):\nWGENerator:MODulation:AM:FREQuency"}, {"Level"=5, "Class Only"=FALSE, "Identifier"="RSRTX_ATTR_WAVEFORM_GENERATOR_AM_MODULATION_DEPTH", "Descriptive Name"="Waveform Generator AM Modulation Depth", "Data Type"=1, "Command"="WGEN:MOD:AM:DEPT", "Access"=2, "Range Table"="", "Read Callback"="", "Write Callback"="", "Supported Models"="", "Instrument Options"="", "Flags"=0, "Help"="Sets the amplitude modulation depth.\n\nAvailable Repeated Capabilities:\nNone\n\nRemote-control command(s):\nWGENerator:MODulation:AM:DEPTh"}, {"Level"=4, "Class Only"=TRUE, "Identifier"="", "Descriptive Name"="FM", "Data Type"=0, "Command"="", "Access"=0, "Range Table"="", "Read Callback"="", "Write Callback"="", "Supported Models"="", "Instrument Options"="", "Flags"=0, "Help"="For frequency modulation (FM), the frequency of the carrier signal is varied according to the modulation signal."}, {"Level"=5, "Class Only"=FALSE, "Identifier"="RSRTX_ATTR_WAVEFORM_GENERATOR_FM_MODULATION_FREQUENCY", "Descriptive Name"="Waveform Generator FM Modulation Frequency", "Data Type"=1, "Command"="WGEN:MOD:FM:FREQ", "Access"=2, "Range Table"="", "Read Callback"="", "Write Callback"="", "Supported Models"="", "Instrument Options"="", "Flags"=0, "Help"="Sets the frequency of the modulation waveform for frequency modulation.\n\nAvailable Repeated Capabilities:\nNone\n\nRemote-control command(s):\nWGENerator:MODulation:FM:FREQuency"}, {"Level"=5, "Class Only"=FALSE, "Identifier"="RSRTX_ATTR_WAVEFORM_GENERATOR_FM_MODULATION_FREQUENCY_DEVIATION", "Descriptive Name"="Waveform Generator FM Modulation Frequency Deviation", "Data Type"=1, "Command"="WGEN:MOD:FM:DEV", "Access"=2, "Range Table"="", "Read Callback"="", "Write Callback"="", "Supported Models"="", "Instrument Options"="", "Flags"=0, "Help"="Sets the frequency deviation, the maximum difference between and FM modulated signal and the carrier signal.\n\nAvailable Repeated Capabilities:\nNone\n\nRemote-control command(s):\nWGENerator:MODulation:FM:DEViation"}, {"Level"=4, "Class Only"=TRUE, "Identifier"="", "Descriptive Name"="ASK", "Data Type"=0, "Command"="", "Access"=0, "Range Table"="", "Read Callback"="", "Write Callback"="", "Supported Models"="", "Instrument Options"="", "Flags"=0, "Help"="For amplitude modulation (AM), the amplitude of the carrier signal is varied according to the modulation signal."}, {"Level"=5, "Class Only"=FALSE, "Identifier"="RSRTX_ATTR_WAVEFORM_GENERATOR_ASK_MODULATION_FREQUENCY", "Descriptive Name"="Waveform Generator ASK Modulation Frequency", "Data Type"=1, "Command"="WGEN:MOD:ASK:FREQ", "Access"=2, "Range Table"="", "Read Callback"="", "Write Callback"="", "Supported Models"="", "Instrument Options"="", "Flags"=0, "Help"="Sets the frequency of the modulation waveform for ASK 
